vi "SLSC Initialize UEGO Calibration Register.vi"(8 "error in (no error)":errorcluster) -> (0 "error out":errorcluster, 3 "Calibrate? Register":refnum<k21>="Calibrate? Register")   [LabVIEW 2014, in "SLSC FPGA Toolkit.lvlib"]
uses:
  SLSC FPGA Toolkit.lvlib
  <vilib>/rvi/DataTransferAndStorage/Container/Common/niFpgaContainerGetUniqueNameForEmu.vi
  <vilib>/rvi/DataTransferAndStorage/Container/Common/niFpgaContainerSetEmuInfo.vi
  <vilib>/rvi/eio/common/nirviEmuReportErrorAndStop.vi
  <vilib>/rvi/LocalResourceManager/LocalResourceManager.xnode
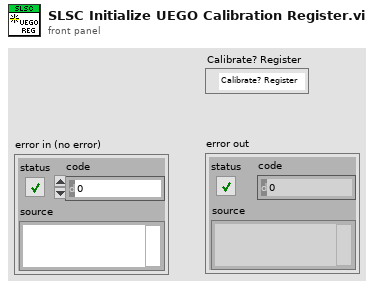
[diagram p1: front panel]
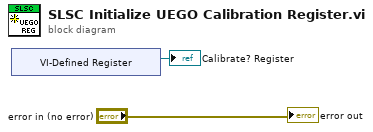
[diagram p0: block diagram]
diagram:
  n1 = xnode "VI-Defined Register"() -> ("Register Out"=→"Calibrate? Register":refnum<k21>)
  "error out" <- "error in (no error)"
